vi "subTimeDelay.vi"(0 "Delay Time (Seconds)":dbl format="%0.2f") -> ()   [LabVIEW 2022 SP3]
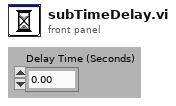
[diagram p1: front panel]
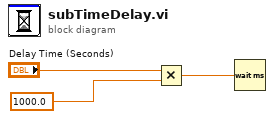
[diagram p0: block diagram]
diagram:
  n1 = Multiply(x="Delay Time (Seconds)", y=1000.0) -> (x*y=w2:dbl)
  n2 = Wait (ms)(milliseconds to wait=w2) -> ()  [unwired: 1 out]
